vi "Append Topic Ref.vi"(8 "error in (no error)":errorcluster, 10 "Topic In":refnum<class "Topic.lvclass">, 11 "TOC in":refnum<class "TOC.lvclass">) -> (0 "error out":errorcluster, 3 "TOC out":refnum<class "TOC.lvclass">)   [LabVIEW 2020, in "TOC.lvclass"]
uses:
  TOC.lvclass
  Topic/Topic.lvclass
  TOC.lvclass/TOC.ctl
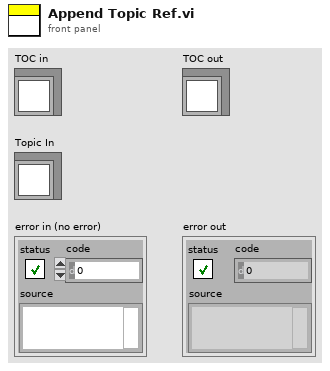
[diagram p1: front panel]
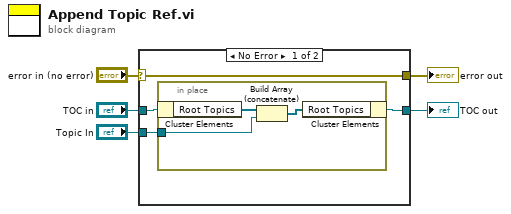
[diagram p0: block diagram]
diagram:
  n1 = case shown="No Error" "error in (no error)" {
    selector: "error in (no error)" -> [w9 w14]
    tunnel: [w9 w14] -> w4
    tunnel: [w7 w13] -> w2
    tunnel: "TOC in" -> [w8 w13]
    tunnel: "Topic In" -> [w6 _]
    frame No Error {
      n2 = in-place {
        in-place-border: w6 -> [w10]
        n3 = in-place-cluster #1(w8) -> ("Root Topics"=w12:refnum<class "Topic.lvclass">[])
        n4 = Build Array (concatenate)(w12, w10) -> (w11:refnum<class "Topic.lvclass">[])
        n5 = in-place-cluster #1("Root Topics"=w11) -> (w7:refnum<class "TOC.lvclass">)
      }
    }
    frame Error {
    }
  }
  "error out" <- w4
  "TOC out" <- w2
